vi "get channels.vi"(11 "Scaling configuration in":refnum<class "Scaling configuration.lvclass">) -> (2 "channels":refnum<class "TBM channel.lvclass">[](array[class]), 3 "Scaling configuration out":refnum<class "Scaling configuration.lvclass">)   [LabVIEW 2013, in "Scaling configuration.lvclass"]
uses:
  Scaling configuration.lvclass
  <vilib>/NI/Tag Bus Module Framework/channel/TBM channel.lvclass
  Scaling configuration.lvclass/Scaling configuration.ctl
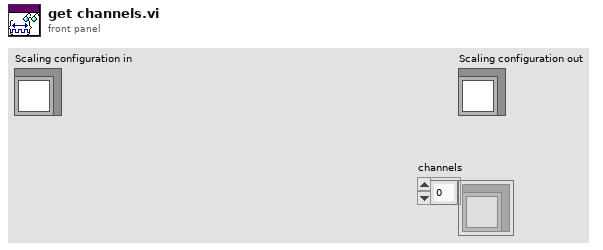
[diagram p1: front panel]
types:
  T1 = typedef "Scaling configuration.lvclass/scale data types.ctl" = enum16{"Double", "Single", "I64", "I32", "I16", "I8", "U64", "U32", "U16", "U8"}
  T2 = cluster{"mappings":cluster{"input channel":refnum<class "TBM channel.lvclass">, "output channel":refnum<class "TBM channel.lvclass">, "input data type":T1, "output data type":T1}[], "name":string}[]
  T3 = cluster{"input channel":refnum<class "TBM channel.lvclass">, "output channel":refnum<class "TBM channel.lvclass">, "input data type":T1, "output data type":T1}[]
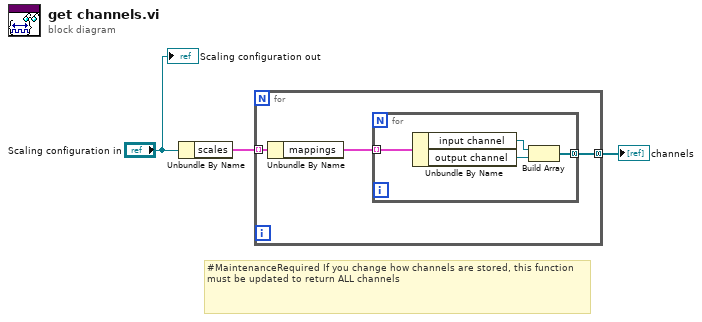
[diagram p0: block diagram]
diagram:
  # "#MaintenanceRequired If you change how channels are stored, this function must be updated to return ALL channels"
  n1 = Unbundle By Name("Scaling configuration in") -> ("scales"=w2:T2)
  n2 = for {
    tunnel: w2 -> [w5] mode=indexing
    tunnel: [w6] -> w1 mode=concatenating
    n3 = Unbundle By Name(w5) -> ("mappings"=w4:T3)
    n4 = for {
      tunnel: w4 -> [w10] mode=indexing
      tunnel: [w7] -> w6 mode=concatenating
      n5 = Unbundle By Name(w10) -> ("input channel"=w9:refnum<class "TBM channel.lvclass">, "output channel"=w8:refnum<class "TBM channel.lvclass">)
      n6 = Build Array(w9, w8) -> (w7:refnum<class "TBM channel.lvclass">[])
    }
  }
  "channels" <- w1
  "Scaling configuration out" <- "Scaling configuration in"
